vi "Bash Escape String.vi"(11 "string in":string) -> (3 "string out":string)   [LabVIEW 2014, in "lvprj2html.lvlib"]
uses:
  lvprj2html.lvlib
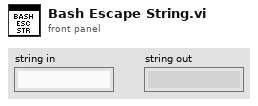
[diagram p1: front panel]
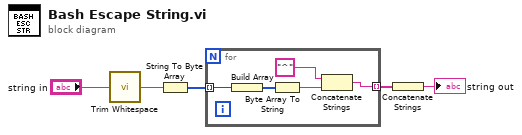
[diagram p0: block diagram]
diagram:
  n1 = call <vilib>:"Trim Whitespace.vi"("string"="string in") -> ("trimmed string"=w2:string)  [unwired: 1 in]
  n2 = String To Byte Array(string=w2) -> (unsigned byte array=w3:u8[])
  n3 = for {
    tunnel: w3 -> [w10] mode=indexing
    tunnel: [w7] -> w4 mode=indexing
    n4 = Build Array(w10) -> (w9:u8[])
    n5 = Byte Array To String(unsigned byte array=w9) -> (string=w8:string)
    n6 = Concatenate Strings("^" ("string"), w8) -> (w7:string)
  }
  n7 = Concatenate Strings(w4) -> (→"string out":string)
